vi "Microwave.vi"(8 "error in (no error)":errorcluster, 11 "Microwave in":refnum<class "Microwave.lvclass">) -> (0 "error out":errorcluster, 3 "Microwave out":refnum<class "Microwave.lvclass">)   [LabVIEW 2017, in "Microwave.lvclass"]
uses:
  Microwave.lvclass
  Global/GPIB Numbers.vi
panel:
  out "Status":string
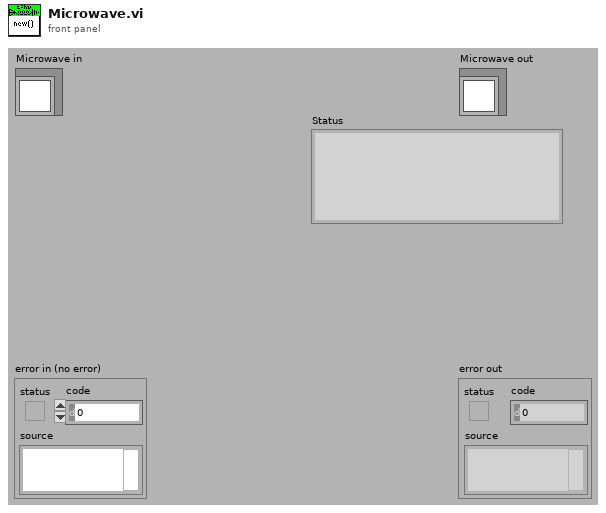
[diagram p1: front panel]
types:
  T1 = typedef "GPIB Type Def.ctl" = cluster{"Name":string, "bus":dbl, "GPIB":dbl, "GPIB as string":string, "byte":i32, "VISA Resource Name":refnum<visa-resource-name>}
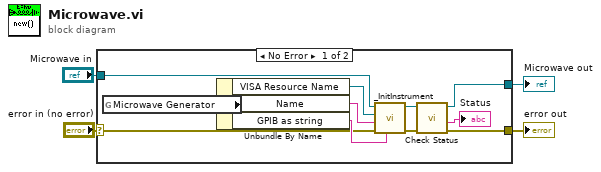
[diagram p0: block diagram]
diagram:
  n1 = case shown="No Error" "error in (no error)" {
    selector: "error in (no error)" -> [w7 w17]
    tunnel: [w6 w17] -> w3
    tunnel: [w8 w16] -> w1
    tunnel: "Microwave in" -> [w9 w16]
    frame No Error {
      n2 = global read "GPIB Numbers.vi" "Microwave Generator"() -> (w13:T1)
      n3 = Unbundle By Name(w13) -> ("VISA Resource Name"=w14:refnum<visa-resource-name>, "Name"=w15:string, "GPIB as string"=w12:string)
      n4 = call-dynamic "_InitInstrument.vi"("GPIB as string"=w12, "error in (no error)"=w7, "Name"=w15, "VISA Resource Name"=w14, "Instrument in"=w9) -> ("error out"=w10:errorcluster, "Instrument out"=w11:refnum<class "Microwave.lvclass">)  [unwired: 1 in, 4 out]
      n5 = call-dynamic "Check Status.vi"("error in (no error)"=w10, "Microwave in"=w11) -> ("error out"=w6:errorcluster, "Status"=→"Status":string, "Microwave out"=w8:refnum<class "Microwave.lvclass">)  [unwired: 7 out]
    }
    frame Error {
    }
  }
  "error out" <- w3
  "Microwave out" <- w1
